vi "Get End Tag.vi"(8 "error in (no error)":errorcluster, 10 "Name":string, 11 "Data Item in":refnum<class "Data Item.lvclass">) -> (0 "error out":errorcluster, 2 "End Tag":string, 3 "Data Item out":refnum<class "Data Item.lvclass">)   [LabVIEW 2026, in "VILab.lvlib" / "Data Item.lvclass"]
uses:
  Data Item.lvclass
  Data Item.lvclass/Data Item.ctl
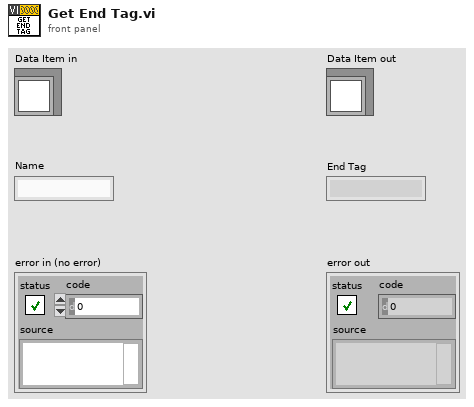
[diagram p1: front panel]
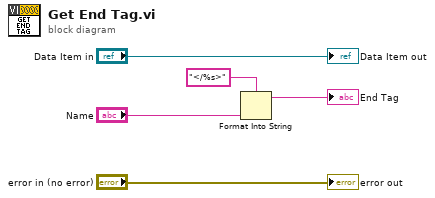
[diagram p0: block diagram]
diagram:
  n1 = Format Into String(format string="</%s>", "Name") -> (resulting string=→"End Tag":string)  [unwired: 2 in, 1 out]
  "error out" <- "error in (no error)"
  "Data Item out" <- "Data Item in"
